vi "Read Point Position Velocity.vi"   [LabVIEW 2011, in "LVH-Leap.lvlib"]
uses:
  LVH-Leap.lvlib
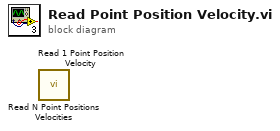
[diagram p0: block diagram]
diagram:
  n1 = call "Read N Point Positions Velocities.vi"() -> ()  [unwired: 8 in, 4 out]
  n2 = call "Read 1 Point Position Velocity.vi"() -> ()  [unwired: 8 in, 4 out]
